vi "Loop_ProtoType Test.vi"() -> ()   [LabVIEW 2017, in "SRX SubSystem.lvlib"]
uses:
  SRX SubSystem.lvlib
  _SHARE ALL/RoboRio Share All/SRX Share All/TypeDefs SRX/Cluster_SRX_General Data.ctl
  _SHARE ALL/RoboRio Share All/SRX Share All/TypeDefs SRX/Cluster_SRX_Common Runtime Data.ctl
  _SHARE ALL/RoboRio Share All/SRX Share All/TypeDefs SRX/Cluster_SRX_Error Calculations.ctl
  _SHARE ALL/RoboRio Share All/SRX Share All/TypeDefs SRX/Cluster_SRX_Voltage Out Data.ctl
  _SHARE ALL/RoboRio Share All/SRX Share All/TypeDefs SRX/Cluster_SRX_Sensor Out Data.ctl
  _SHARE ALL/RoboRio Share All/SRX Share All/TypeDefs SRX/Cluster_SRX_Sensor Quad Data.ctl
  _SHARE ALL/RoboRio Share All/SRX Share All/TypeDefs SRX/Cluster_SRX_Analog In Data.ctl
  _SHARE ALL/RoboRio Share All/SRX Share All/TypeDefs SRX/Cluster_SRX_PWM Sensor Data.ctl
  _SHARE ALL/RoboRio Share All/SRX Share All/TypeDefs SRX/Cluster_SRX_F and R Limit Indicators.ctl
  _SHARE ALL/RoboRio Share All/SRX Share All/TypeDefs SRX/Cluster_SRX_Faults.ctl
  _SHARE ALL/RoboRio Share All/SRX Share All/TypeDefs SRX/Cluster_SRX_Config Voltage Output.ctl
  System Drivers/Phoenix-LabVIEW/Motor Controller/Controls/CTRE_Phoenix_MotorControl_NeutralMode.ctl
  _SHARE ALL/RoboRio Share All/SRX Share All/TypeDefs SRX/Cluster_SRX_Forward and Reverse.ctl
  _SHARE ALL/RoboRio Share All/SRX Share All/TypeDefs SRX/Cluster_SRX_Current Config.ctl
  _SHARE ALL/RoboRio Share All/SRX Share All/TypeDefs SRX/Cluster_SRX_Config Soft Limits.ctl
  _SHARE ALL/RoboRio Share All/SRX Share All/TypeDefs SRX/Cluster_SRX_Config Hard Limits.ctl
  System Drivers/Phoenix-LabVIEW/Motor Controller/Controls/CTRE_Phoenix_MotorControl_LimitSwitchNormal.ctl
  _SHARE ALL/RoboRio Share All/SRX Share All/TypeDefs SRX/Cluster_SRX_PIDF.ctl
  _SHARE ALL/RoboRio Share All/SRX Share All/TypeDefs SRX/Cluster_SRX_Motion Magic Config Data.ctl
  _SHARE ALL/RoboRio Share All/SRX Share All/TypeDefs SRX/Cluster_SRX_Mode and Value.ctl
  System Drivers/Phoenix-LabVIEW/Motor Controller/Controls/CTRE_Phoenix_MotorControl_ControlMode.ctl
  _SHARE ALL/RoboRio Share All/SRX Share All/TypeDefs SRX/ENUM_SRX_Reset Select.ctl
  _SHARE ALL/RoboRio Share All/SRX Share All/TypeDefs SRX/Cluster_SRX_Sensor Config.ctl
  System Drivers/Phoenix-LabVIEW/Motor Controller/Controls/CTRE_Phoenix_MotorControl_FeedbackDevice.ctl
  System Drivers/Phoenix-LabVIEW/Controls/CTRE_Phoenix_Params.ctl
  ENUM_SM_State.ctl
  <vilib>/Rock Robotics/WPI/MotorControl/WPI_MotorControlDeviceRef.ctl
  <vilib>/Rock Robotics/WPI/MotorControl/WPI_MotorControlType.ctl
  <vilib>/Rock Robotics/SystemInterfaces/DIO/FPGA_DIOPWMChannel.ctl
  <vilib>/Rock Robotics/WPI/PWM/WPI_PWMDeadband.ctl
  <vilib>/Rock Robotics/SystemInterfaces/DIO/FPGA_DIOChannel.ctl
  ENUM_SM_Action.ctl
  _SHARE ALL/Global Share All/Global_STOP.vi
  Global_CMD.vi
panel:
  out "Encoder Data":enum32{"PWM", "Analog", "Quad"}(tab)
  out "PWM Data":T1
  out "Analog Sensor Data":T2
  out "Quad Sensor Data Out":T3
  in  "TYPE":bool
  in  "Master Invert":bool
  in  "Follow Tab":T4(tab)
  in  "Follow1 Invert":bool
  in  "Follower 1":u8=14
  in  "FB Invert":bool
  in  "FA Invert":bool
  in  "Follower A":u8=14
  in  "Follower B":u8=14
  in  "Clear Error":bool
  out "Waveform Chart":cluster{"Value":dbl, "Pos":i32, "Vel":i32}(graph)
  out "Mode And Value":T5 {"Mode" items=["PercentOutput"=0, "Position"=1, "Velocity"=2, "Current"=3, "Follower"=5, "MotionProfile"=6, "MotionMagic"=7, "MotionMagicArc"=8, "MotionProfileArc"=10, "Disabled"=15]}
  out "Current Error":errorcluster
  in  "Master ID":u8=14
  in  "Tab":enum32{"Config", "Set", "Settings"}(tab)
  in  "Set Data":bool
  in  "Config":T7(tab)
  in  "Voltage Out Config":T8={"Invert?"=FALSE, "Neutral Mode"=enum."Override to Brake", "Deadband (-1to1)"=0.02, "Ramp Time Off to Full (S)"=0.01, "Peak  (-1to1)"={"Forward"=1.0, "Reverse"=-1.0}, "Nominal  (-1to1)"={"Forward"=0.0, "Reverse"=0.0}}
  in  "Sensor Config":T11={"Feedback Device"=enum."None", "PhaseSensor"=TRUE}
  in  "Current Out Config":T13
  in  "Soft Limits (Units)":T14={"Max"=200000, "Min"=-200000, "Max Enable"=TRUE, "Min Enable"=TRUE}
  in  "Hard Limits":T15
  in  "Motion Magic Config Data":T17
  in  "AllowableClosedLoopError":i32=300
  in  "Maximum I-Acc":dbl
  in  "SlotIdx":i32
  in  "Use Slot":bool
  in  "Target Slot":i32
  in  "Reset":bool
  in  "Reset Select":T18
  in  "Set PIDF 1":bool
  in  "PIDF 0":T19={"P"=0.02, "I"=0.0, "D"=6.0, "F"=0.0, "I Zone"=3000.0}
  in  "PIDF 1":T19
  in  "Set PIDF 0":bool
  in  "Enable":bool
  in  "Param Select":T20[](array[typedef]) items=["eOnBoot_BrakeMode"=31, "eQuadFilterEn"=91, "eQuadIdxPolarity"=108, "eClearPositionOnIdx"=100, "eMotionProfileHasUnderrunErr"=119, "eMotionProfileTrajectoryPointDurationMs"=120, "eClearPosOnLimitF"=144, "eClearPosOnLimitR"=145, "eStatusFramePeriod"=300, "eOpenLoopRamp"=301, "eClosedLoopRamp"=302, "eNeutralDeadband"=303, "ePeakPosOutput"=305, "eNominalPosOutput"=306, "ePeakNegOutput"=307, "eNominalNegOutput"=308, "eProfileParamSlot_P"=310, "eProfileParamSlot_I"=311, "eProfileParamSlot_D"=312, "eProfileParamSlot_F"=313, "eProfileParamSlot_IZone"=314, "eProfileParamSlot_AllowableErr"=315, "eProfileParamSlot_MaxIAccum"=316, "eClearPositionOnLimitF"=320, "eClearPositionOnLimitR"=321, "eClearPositionOnQuadIdx"=322, "eSampleVelocityPeriod"=325, "eSampleVelocityWindow"=326, "eFeedbackSensorType"=330, "eSelectedSensorPosition"=331, "eFeedbackNotContinuous"=332, "eRemoteSensorSource"=333, "eRemoteSensorDeviceID"=334, "eSensorTerm"=335, "eRemoteSensorClosedLoopDisableNeutralOnLOS"=336, "eForwardSoftLimitThreshold"=340, "eReverseSoftLimitThreshold"=341, "eForwardSoftLimitEnable"=342, "eReverseSoftLimitEnable"=343, "eNominalBatteryVoltage"=350, "eBatterVoltageFilterSize"=351, "eContinuousCurrentLimitAmps"=360, "eContinuousCurrentLimitMs"=361, "ePeakCurrentLimitAmps"=362, "eClosedLoopIAccum"=370, "eCustomParam"=380, "eStickyFaults"=390, "eAnalogPosition"=400, "eQuadraturePosition"=401, "ePulseWidthPosition"=402, "eMotMag_Accel"=410, "eMotMag_VelCruise"=411, "eLimitSwitchSource"=421, "eLimitSwitchNormClosedAndDis"=422, "eLimitSwitchDisabledNeutralOnLOS"=423, "eLimitSwitchRemoteDevID"=424]
  in  "Read Info":bool
  out "Value Array":dbl[](array[numeric])
  out "Last Error Code":i32
  out "Faults Out":T21
  out "Hard Limits":T22
  out "Last Error":errorcluster
  out "Common Runtime Data Out":T23 {"Temp" format="%.1f"; "Voltage"."Bus" format="%.3f"; "Voltage"."Output" format="%.3f"; "Voltage"."Percent" format="%.3f"; "Current" format="%.2f"}
  out "Device Info":T27
  out "Cycle Time (S)":dbl format="%.3g"
  # "VICTOR"
  # "TALON"
  # "C"
  # "Units"
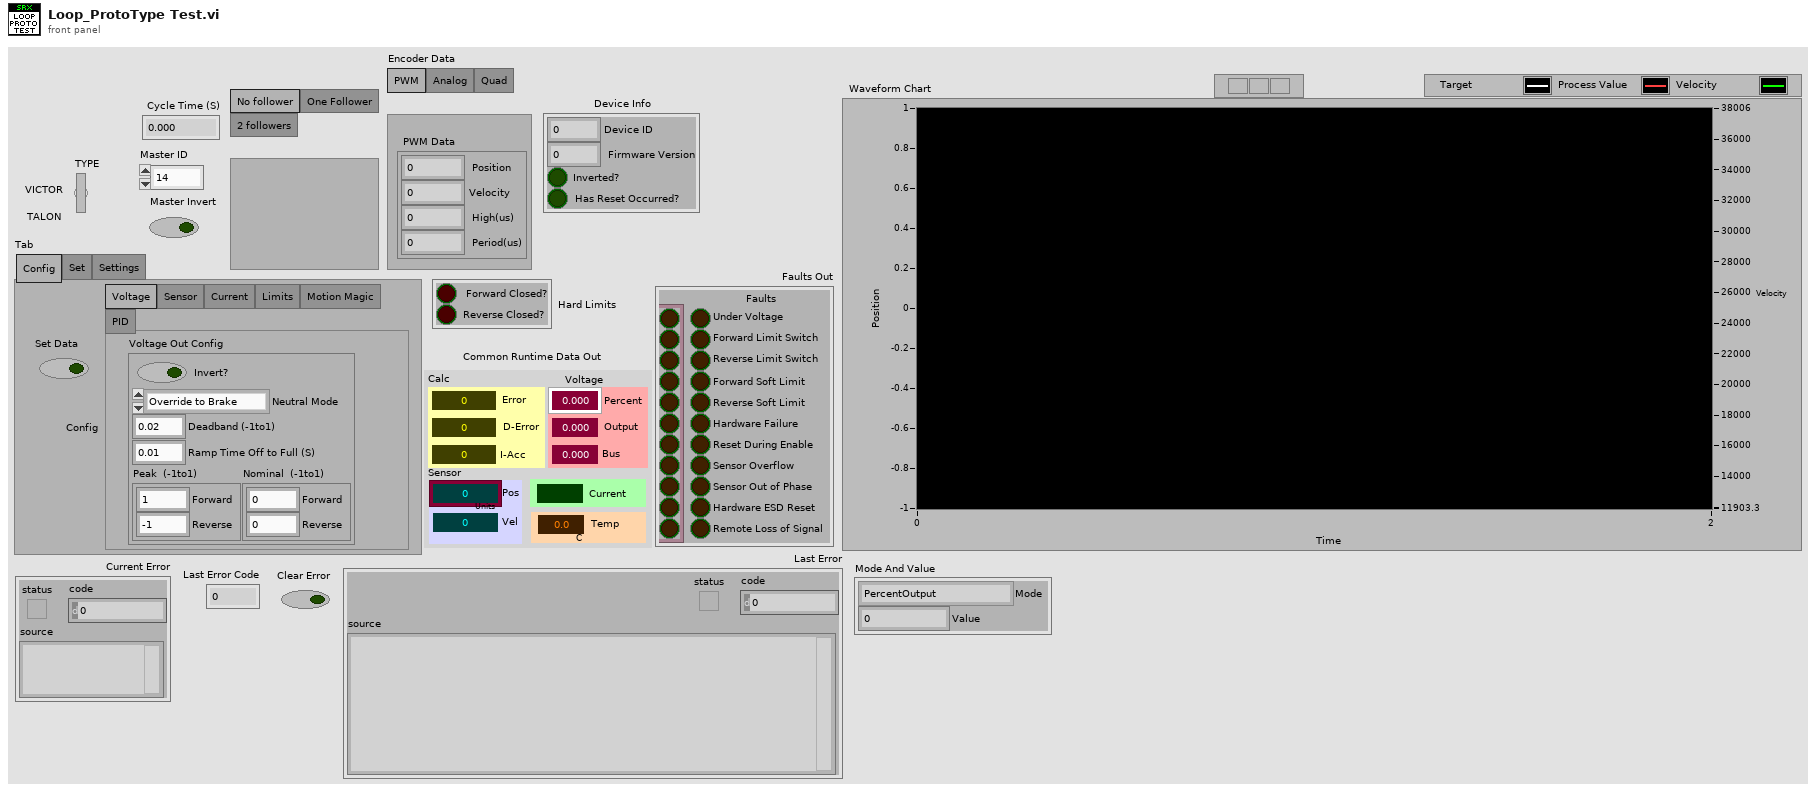
[diagram p1: front panel]
types:
  T1 = typedef "Cluster_SRX_PWM Sensor Data.ctl" = cluster{"Position":i32, "Velocity":i32, "High(us)":i32, "Period(us)":i32}
  T2 = typedef "Cluster_SRX_Analog In Data.ctl" = cluster{"WithOv":i32, "Raw":i32, "Velocity":i32}
  T3 = typedef "Cluster_SRX_Sensor Quad Data.ctl" = cluster{"Position":i32, "Velocity":i32, "Quad A Pin":bool, "Quad B Pin":bool, "Quad Idx Pin":bool}
  T4 = enum32{"No follower", "One Follower", "2 followers"}
  T5 = typedef "Cluster_SRX_Mode and Value.ctl" = cluster{"Mode":T6, "Value":dbl}
  T6 = typedef "CTRE_Phoenix_MotorControl_ControlMode.ctl" = u16
  T7 = enum32{"Voltage", "Sensor", "Current", "Limits", "Motion Magic", "PID"}
  T8 = typedef "Cluster_SRX_Config Voltage Output.ctl" = cluster{"Invert?":bool, "Neutral Mode":T9, "Deadband (-1to1)":dbl, "Ramp Time Off to Full (S)":dbl, "Peak  (-1to1)":T10, "Nominal  (-1to1)":T10}
  T9 = typedef "CTRE_Phoenix_MotorControl_NeutralMode.ctl" = enum8{"EEPROMSetting", "Override to Coast", "Override to Brake"}
  T10 = typedef "Cluster_SRX_Forward and Reverse.ctl" = cluster{"Forward":dbl, "Reverse":dbl}
  T11 = typedef "Cluster_SRX_Sensor Config.ctl" = cluster{"Feedback Device":T12, "PhaseSensor":bool}
  T12 = typedef "CTRE_Phoenix_MotorControl_FeedbackDevice.ctl" = enum16{"None", "QuadEncoder", "Analog", "Tachometer", "Pulse Width Encoded Position", "Sensor Sum (S0 + S1)", "Sensor Difference (D0 - D1)", "Remote Source 0", "Remote Source 1", "Software Emulated"}
  T13 = typedef "Cluster_SRX_Current Config.ctl" = cluster{"Enable Current Limit?":bool, "Peak Current (Amps)":i32, "Peak Current Maximum Duration (ms)":i32, "Continuous Current Limit (Amps)":i32}
  T14 = typedef "Cluster_SRX_Config Soft Limits.ctl" = cluster{"Max":i32, "Min":i32, "Max Enable":bool, "Min Enable":bool}
  T15 = typedef "Cluster_SRX_Config Hard Limits.ctl" = cluster{"Fwd Enable":bool, "Rev Enable":bool, "Fwd NO-NC":T16, "Rev NO-NC":T16}
  T16 = typedef "CTRE_Phoenix_MotorControl_LimitSwitchNormal.ctl" = enum16{"Normally Open", "Normally Closed", "Disabled"}
  T17 = typedef "Cluster_SRX_Motion Magic Config Data.ctl" = cluster{"Cruise Velocity":i32, "Acceleration":i32}
  T18 = typedef "ENUM_SRX_Reset Select.ctl" = enum16{"None", "Sensor", "I-Accum", "Sticky Faults", "ALL"}
  T19 = typedef "Cluster_SRX_PIDF.ctl" = cluster{"P":dbl, "I":dbl, "D":dbl, "F":dbl, "I Zone":dbl}
  T20 = typedef "CTRE_Phoenix_Params.ctl" = u16
  T21 = typedef "Cluster_SRX_Faults.ctl" = cluster{"Sticky":cluster{"Under Voltage":bool, "Forward Limit Switch":bool, "Reverse Limit Switch":bool, "Forward Soft Limit":bool, "Reverse Soft Limit":bool, "Hardware Failure":bool, "Reset During Enable":bool, "Sensor Overflow":bool, "Sensor Out of Phase":bool, "Hardware ESD Reset":bool, "Remote Loss of Signal":bool}, "Faults":cluster{"Under Voltage":bool, "Forward Limit Switch":bool, "Reverse Limit Switch":bool, "Forward Soft Limit":bool, "Reverse Soft Limit":bool, "Hardware Failure":bool, "Reset During Enable":bool, "Sensor Overflow":bool, "Sensor Out of Phase":bool, "Hardware ESD Reset":bool, "Remote Loss of Signal":bool}}
  T22 = typedef "Cluster_SRX_F and R Limit Indicators.ctl" = cluster{"Forward Closed?":bool, "Reverse Closed?":bool}
  T23 = typedef "Cluster_SRX_Common Runtime Data.ctl" = cluster{"Calc":T24, "Voltage ":T25, "Sensor":T26, "Current":dbl, "Temp":dbl}
  T24 = typedef "Cluster_SRX_Error Calculations.ctl" = cluster{"Error":i32, "D-Error":dbl, "I-Acc":dbl}
  T25 = typedef "Cluster_SRX_Voltage Out Data.ctl" = cluster{"Percent":dbl, "Output":dbl, "Bus":dbl}
  T26 = typedef "Cluster_SRX_Sensor Out Data.ctl" = cluster{"Pos":i32, "Vel":i32}
  T27 = typedef "Cluster_SRX_General Data.ctl" = cluster{"Device ID":i32, "Firmware Version":i32, "Inverted?":bool, "Has Reset Occurred?":bool}
  T28 = typedef "SRX SubSystem.lvlib/ENUM_SM_Action.ctl" = enum16{"No Action", "Reset Time", "Reset All", "Set Mode and Value", "Set PIDF Slot 0", "Set PIDF Slot 1", "Reset", "Set PID Slot", "Create Master SRX", "Create Followers SRX"}
  T29 = typedef "WPI_MotorControlDeviceRef.ctl" = cluster{"DeviceStatus":errorcluster, "Type":T30, "PWM":cluster{"PWM Channel":T31, "DeadBand":T32}, "CAN":cluster{"Device Number":u8, "SetOutput VI Ref":variant, "GetOutput VI Ref":variant, "Enable VI Ref":variant, "Disable VI Ref":variant, "Data":variant}, "Invert":bool, "DIO PWM":cluster{"PWM \"Enable\" Channel":T31, "DIOChannel":T33, "PWM Rate":dbl}}
  T30 = typedef "WPI_MotorControlType.ctl" = enum16{"PWM", "CAN", "DIO PWM"}
  T31 = typedef "FPGA_DIOPWMChannel.ctl" = enum8{"PWM 0", "PWM 1", "PWM 2", "PWM 3", "PWM 4", "PWM 5", "PWM 6", "PWM 7", "PWM 8", "PWM 9", "PWM MXP 0", "PWM MXP 1", "PWM MXP 2", "PWM MXP 3", "PWM MXP 4", "PWM MXP 5", "PWM MXP 6", "PWM MXP 7", "PWM MXP 8", "PWM MXP 9", "Invalid"}
  T32 = typedef "WPI_PWMDeadband.ctl" = cluster{"Name":string, "maxPositivePwm":i32, "minPositivePwm":i32, "centerPwm":i32, "maxNegativePwm":i32, "minNegativePwm":i32, "angularRange":u16}
  T33 = typedef "FPGA_DIOChannel.ctl" = enum8{"DIO 0", "DIO 1", "DIO 2", "DIO 3", "DIO 4", "DIO 5", "DIO 6", "DIO 7", "DIO 8", "DIO 9", "DIO MXP 0", "DIO MXP 1", "DIO MXP 2", "DIO MXP 3", "DIO MXP 4", "DIO MXP 5", "DIO MXP 6", "DIO MXP 7", "DIO MXP 8", "DIO MXP 9", "DIO MXP 10", "DIO MXP 11", "DIO MXP 12", "DIO MXP 13", "DIO MXP 14", "DIO MXP 15", "SPI Port CS1", "SPI Port CS2", "SPI Port CS3", "SPI Port MISO", "SPI Port MOSI", "Invalid"}
  T34 = typedef "SRX SubSystem.lvlib/ENUM_SM_State.ctl" = enum16{"Startup", "Idle", "Shutdown"}
  T35 = cluster{"State":T34, "Previous State":T34, "Current Time":timestamp, "Previous Time":timestamp, "Start Time":timestamp, "Target Time (ms)":u32, "Cycle Time(S)":dbl, "SRX Ref":T29, "Error":errorcluster, "SRX Mode":T5, "Reset Select":T18, "Target Slot":i32, "PIDF":T19, "Sensor Config":T11}
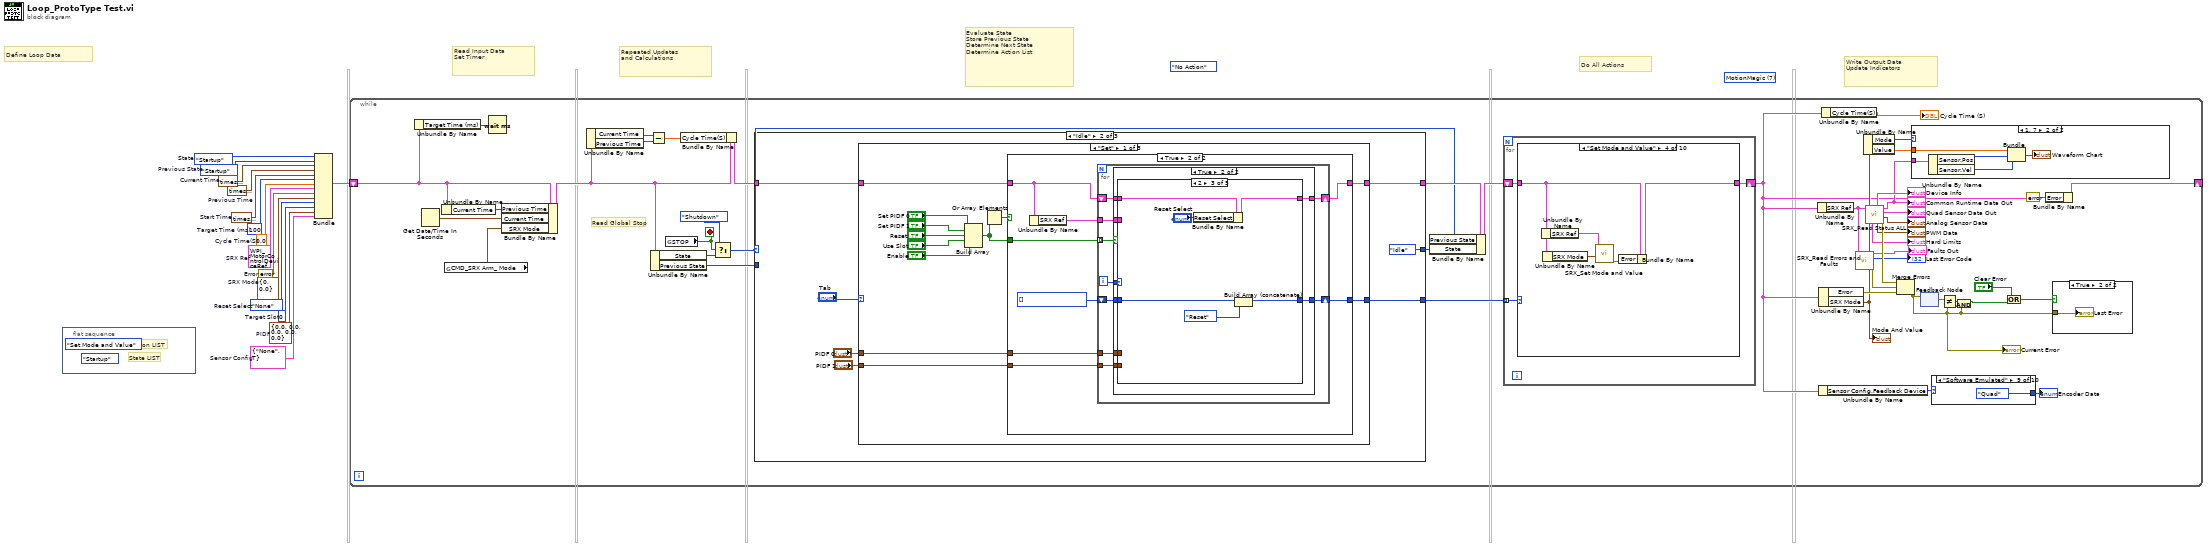
[diagram p0: block diagram]
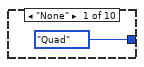
[diagram p2: hidden frame]
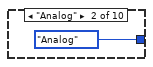
[diagram p3: hidden frame]
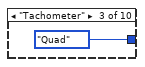
[diagram p4: hidden frame]
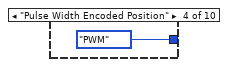
[diagram p5: hidden frame]
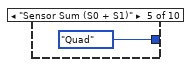
[diagram p6: hidden frame]
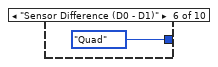
[diagram p7: hidden frame]
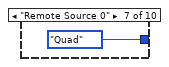
[diagram p8: hidden frame]
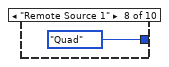
[diagram p9: hidden frame]
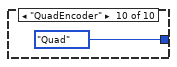
[diagram p10: hidden frame]
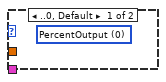
[diagram p11: hidden frame]
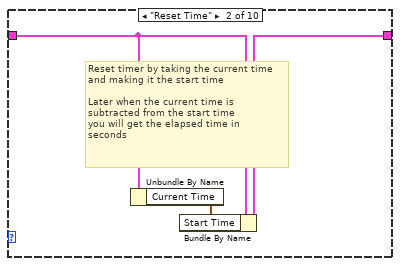
[diagram p14: hidden frame]
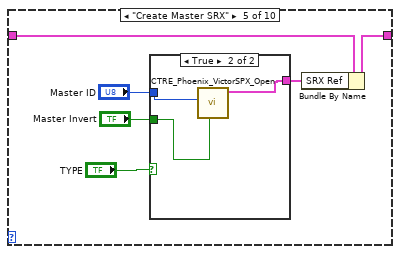
[diagram p16: hidden frame]
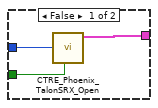
[diagram p17: hidden frame]
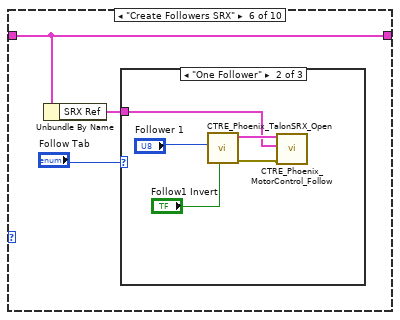
[diagram p18: hidden frame]
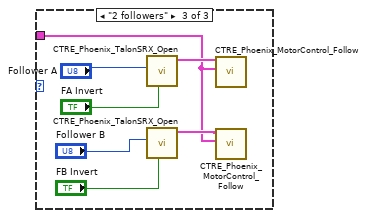
[diagram p20: hidden frame]
diagram:
  (unwired) ENUM_SM_Action."No Action" ("Action")
  w1 = T11 {"Feedback Device"=enum."None", "PhaseSensor"=TRUE}  # Sensor Config
  (unwired) T6 7 items=["PercentOutput"=0, "Position"=1, "Velocity"=2, "Current"=3, "Follower"=5, "MotionProfile"=6, "MotionMagic"=7, "MotionMagicArc"=8, "MotionProfileArc"=10, "Disabled"=15] ("Mode")
  w3 = T19 {"P"=0.0, "I"=0.0, "D"=0.0, "F"=0.0, "I Zone"=0.0}  # PIDF
  w4 = 0  # Target Slot
  w5 = ENUM_SRX_Reset_Select."None"  # Reset Select
  w6 = T5 {"Mode"=0, "Value"=0.0}  # SRX Mode
  w7 = errorcluster {"status"=FALSE, "code"=0, "source"=""}  # Error
  w8 = T29 {"DeviceStatus"={"status"=FALSE, "code"=0, "source"=""}, "Type"=enum."PWM", "PWM"={"PWM Channel"=enum."Invalid", "DeadBand"={"Name"="", "maxPositivePwm"=0, "minPositivePwm"=0, "centerPwm"=0, "maxNegativePwm"=0, "minNegativePwm"=0, "angularRange"=0}}, "CAN"={"Device Number"=0, "SetOutput VI Ref"=variant(enum8{"Percent VBus", "Current", "Speed", "Position", "Voltage"} enum."Percent VBus"), "GetOutput VI Ref"=variant(refnum<k1> refnum), "Enable VI Ref"=variant(dbl 12.0), "Disable VI Ref"=variant(enum8{"Percent VBus", "Speed", "Position", "Slave", "Unchanged / Invalid", "Voltage Compensation", "Current", "Motion Profile"} enum."Percent VBus"), "Data"=variant}, "Invert"=FALSE, "DIO PWM"={"PWM \"Enable\" Channel"=enum."Invalid", "DIOChannel"=enum."Invalid", "PWM Rate"=0.0}}  # SRX Ref
  w9 = 0.0  # Cycle Time(S)
  w10 = ENUM_SM_State."Startup"  # Previous State
  w11 = timestamp(0 s since 1904-01-01)  # Previous Time
  w12 = u32 100  # Target Time (ms)
  w13 = timestamp(0 s since 1904-01-01)  # Start Time
  w14 = timestamp(0 s since 1904-01-01)  # Current Time
  w15 = ENUM_SM_State."Startup"  # State
  # "Define Loop Data"
  # "Repeated Updates\nand Calculations"
  # "Read Input Data\nSet Timer"
  # "Evaluate State\nStore Previous State\nDetermine Next State\nDetermine Action List"
  # "Do All Actions"
  # "Write Output Data\nUpdate Indicators"
  n1 = flat-sequence {
    frame #0 {
      (unwired) ENUM_SM_State."Startup" ("State")
      (unwired) ENUM_SM_Action."Set Mode and Value" ("Action")
      # "State LIST"
      # "Action LIST"
    }
  }
  n2 = Bundle("State"=w15, "Previous State"=w10, "Current Time"=w14, "Previous Time"=w11, "Start Time"=w13, "Target Time (ms)"=w12, "Cycle Time(S)"=w9, "SRX Ref"=w8, "Error"=w7, "SRX Mode"=w6, "Reset Select"=w5, "Target Slot"=w4, "PIDF"=w3, "Sensor Config"=w1) -> (w2:T35)  [unwired: 1 in]
  n3 = while {
    shift-right: [w26] -> _
    shift-left: w2 -> [w52]
    stop <- w57 stop-if-true
    # "Read Global Stop"
    n4 = Unbundle By Name(w52) -> ("Target Time (ms)"=w54:u32)
    n5 = Get Date/Time In Seconds() -> (seconds since 1Jan1904=w61:timestamp)
    n6 = Unbundle By Name(w52) -> ("Current Time"=w53:timestamp)
    n7 = global read "Global_CMD.vi" "CMD_SRX Arm_ Mode"() -> (w42:T5)
    n8 = Wait (ms)(milliseconds to wait=w54) -> ()  [unwired: 1 out]
    n9 = Bundle By Name(cluster=w52, "Previous Time"=w53, "Current Time"=w61, "SRX Mode"=w42) -> (w46:T35)
    n10 = Unbundle By Name(w46) -> ("Current Time"=w47:timestamp, "Previous Time"=w48:timestamp)
    n11 = Subtract(x=w47, y=w48) -> (x-y=w44:dbl)
    n12 = Unbundle By Name(w46) -> ("State"=w55:T34, "Previous State"=w51:T34)
    n13 = global read "Global_STOP.vi" "STOP"() -> (w57:bool)
    n14 = Bundle By Name(cluster=w46, "Cycle Time(S)"=w44) -> (w45:T35)
    n15 = Select(t=ENUM_SM_State."Shutdown" ("State"), s=w57, f=w55) -> (s? t:f=w50:T34)
    n16 = case shown="\"Idle\"" w50 {
      tunnel: w45 -> [w140 w148 w275]
      tunnel: [w140 w147 w275] -> w59
      tunnel: [ENUM_SM_State."Idle" ("State") ENUM_SM_State."Idle" ("State") ENUM_SM_State."Shutdown" ("State")] -> w58
      tunnel: [w142 w143 w273] -> w43
      tunnel: w51 -> [_ _ _]
      frame "Startup" {
        w142 = T28[] [enum."Reset Time", enum."Create Master SRX", enum."Create Followers SRX"] items=["No Action", "Reset Time", "Reset All", "Set Mode and Value", "Set PIDF Slot 0", "Set PIDF Slot 1", "Reset", "Set PID Slot", "Create Master SRX", "Create Followers SRX"] ("Actions")
        # "E"
      }
      frame "Idle" {
        n17 = case shown="\"Set\"" "Tab" {
          tunnel: w148 -> [w155 w220 w232]
          tunnel: [w154 w220 w231] -> w147
          tunnel: "PIDF 0" -> [w152 _ w230]
          tunnel: "PIDF 1" -> [w151 _ w227]
          tunnel: [w150 _ _] -> w143
          frame "Set" {
            n18 = Build Array("Set PIDF 0", "Set PIDF 1", "Reset", "Use Slot", "Enable") -> (w153:bool[])
            n19 = Or Array Elements(Boolean array=w153) -> (logical OR=w156:bool)
            n20 = case shown="True" w156 {
              tunnel: w155 -> [w162 w166]
              tunnel: [w162 w165] -> w154
              tunnel: w153 -> [_ w170]
              tunnel: w152 -> [_ w168]
              tunnel: w151 -> [_ w167]
              tunnel: [_ w163] -> w150
              frame False {
              }
              frame True {
                w164 = T28[] [] items=["No Action", "Reset Time", "Reset All", "Set Mode and Value", "Set PIDF Slot 0", "Set PIDF Slot 1", "Reset", "Set PID Slot", "Create Master SRX", "Create Followers SRX"] ("Actions")
                n21 = Unbundle By Name(w166) -> ("SRX Ref"=w169:T29)
                n22 = for {
                  tunnel: w170 -> [w179] mode=indexing
                  tunnel: w169 -> [w178]
                  tunnel: w168 -> [w176]
                  tunnel: w167 -> [w175]
                  shift-right: [w173] -> w165
                  shift-left: w166 -> [w174]
                  shift-right: [w171] -> w163
                  shift-left: w164 -> [w172]
                  i -> [w177]
                  n23 = case shown="True" w179 {
                    tunnel: w178 -> [_ w188]
                    tunnel: w177 -> [_ w189]
                    tunnel: w176 -> [_ w187]
                    tunnel: w175 -> [_ w186]
                    tunnel: w174 -> [w181 w185]
                    tunnel: [w181 w184] -> w173
                    tunnel: w172 -> [w180 w183]
                    tunnel: [w180 w182] -> w171
                    frame False {
                    }
                    frame True {
                      n24 = case shown="2" w189 {
                        tunnel: w188 -> [_ _ _ _ _]
                        tunnel: w187 -> [w190 _ _ _ _]
                        tunnel: w186 -> [_ w196 _ _ _]
                        tunnel: w185 -> [w192 w198 w204 w213 w216]
                        tunnel: [w191 w197 w203 w212 w216] -> w184
                        tunnel: w183 -> [w195 w201 w207 w210 w217]
                        tunnel: [w194 w200 w206 w209 w215] -> w182
                        frame ..0 {
                          n25 = Bundle By Name(cluster=w192, "PIDF"=w190) -> (w191:T35)
                          n26 = Build Array (concatenate)(w195, ENUM_SM_Action."Set PIDF Slot 0" ("Action")) -> (w194:T28[])
                        }
                        frame 1 {
                          n27 = Bundle By Name(cluster=w198, "PIDF"=w196) -> (w197:T35)
                          n28 = Build Array (concatenate)(w201, ENUM_SM_Action."Set PIDF Slot 1" ("Action")) -> (w200:T28[])
                        }
                        frame 2 {
                          n29 = Bundle By Name(cluster=w204, "Reset Select"="Reset Select") -> (w203:T35)
                          n30 = Build Array (concatenate)(w207, ENUM_SM_Action."Reset" ("Action")) -> (w206:T28[])
                        }
                        frame 3 {
                          n31 = Bundle By Name(cluster=w213, "Target Slot"="Target Slot") -> (w212:T35)
                          n32 = Build Array (concatenate)(w210, ENUM_SM_Action."Set PID Slot" ("Action")) -> (w209:T28[])
                        }
                        frame 4.. {
                          n33 = Build Array (concatenate)(w217, ENUM_SM_Action."Set Mode and Value" ("Action")) -> (w215:T28[])
                        }
                      }
                    }
                  }
                }
              }
            }
          }
          frame "Settings" {
            n34 = Unbundle By Name(w220) -> ("SRX Ref"=w219:T29)
            n35 = case shown="True" "Read Info" {
              tunnel: w219 -> [_ w223]
              frame False {
              }
              frame True {
                n36 = for {
                  tunnel: w223 -> [w226]
                  tunnel: "Param Select" -> [w225] mode=indexing
                  tunnel: [w224] -> w221 mode=indexing
                  n37 = call "CTRE_Phoenix_MotorControl_ConfigGetParameter.vi"("Parameter"=w225, "PhoenixMotorControlDevRef"=w226) -> ("value"=w224:dbl)  [unwired: 7 in, 2 out]
                }
                "Value Array" <- w221
              }
            }
          }
          frame "Config" {
            n38 = case shown="True" "Set Data" {
              tunnel: w232 -> [w233 w237]
              tunnel: [w233 w236] -> w231
              tunnel: w230 -> [_ w238]
              tunnel: "Config" -> [_ w235]
              tunnel: w227 -> [_ w234]
              frame False {
              }
              frame True {
                n39 = case shown="\"Voltage\"" w235 {
                  tunnel: w238 -> [_ _ _ _ _ w272]
                  tunnel: w237 -> [w243 w246 w252 w258 w264 w271]
                  tunnel: [w242 w245 w251 w257 w263 w270] -> w236
                  tunnel: w234 -> [_ _ _ _ _ _]
                  frame "Voltage" {
                    n40 = Unbundle By Name(w243) -> ("SRX Ref"=w239:T29)
                    n41 = call "SRX_Config Voltage Output.vi"("Output Config"="Voltage Out Config", "PhoenixMotorControlDevRef"=w239) -> ("Error Out"=w241:errorcluster)  [unwired: 8 in, 1 out]
                    n42 = Bundle By Name(cluster=w243, "Error"=w241) -> (w242:T35)
                  }
                  frame "Sensor" {
                    n43 = Unbundle By Name(w246) -> ("SRX Ref"=w247:T29)
                    n44 = Bundle By Name(cluster=w246, "Sensor Config"="Sensor Config") -> (w245:T35)
                    n45 = call "SRX_Config Sensor.vi"("Sensor Config"="Sensor Config", "PhoenixMotorControlDevRef"=w247) -> ()  [unwired: 8 in, 2 out]
                  }
                  frame "Current" {
                    n46 = Unbundle By Name(w252) -> ("SRX Ref"=w250:T29)
                    n47 = call "SRX_Config Current Output.vi"("Current Config Data"="Current Out Config", "PhoenixMotorControlDevRef"=w250) -> ("Error Out"=w249:errorcluster)  [unwired: 8 in, 1 out]
                    n48 = Bundle By Name(cluster=w252, "Error"=w249) -> (w251:T35)
                  }
                  frame "Limits" {
                    n49 = Unbundle By Name(w258) -> ("SRX Ref"=w256:T29)
                    n50 = call "SRX_Config Soft Limits.vi"("Soft Limits (Units)"="Soft Limits (Units)", "PhoenixMotorControlDevRef"=w256) -> ("PhoenixMotorControlDevRef Out"=w259:T29)  [unwired: 8 in, 1 out]
                    n51 = call "SRX_Config Hard Limit Switches.vi"("Hard Limits"="Hard Limits", "PhoenixMotorControlDevRef"=w259) -> ("Error Out"=w255:errorcluster)  [unwired: 8 in, 1 out]
                    n52 = Bundle By Name(cluster=w258, "Error"=w255) -> (w257:T35)
                  }
                  frame "Motion Magic" {
                    n53 = Unbundle By Name(w264) -> ("SRX Ref"=w262:T29)
                    n54 = call "SRX_Config Motion Magic.vi"("Motion Magic Config Data"="Motion Magic Config Data", "PhoenixMotorControlDevRef"=w262) -> ("Error Out"=w261:errorcluster)  [unwired: 8 in, 1 out]
                    n55 = Bundle By Name(cluster=w264, "Error"=w261) -> (w263:T35)
                  }
                  frame "PID" {
                    n56 = Unbundle By Name(w271) -> ("SRX Ref"=w268:T29)
                    n57 = call "SRX_Config PID Closed Loop.vi"("AllowableClosedLoopError"="AllowableClosedLoopError", "SlotIdx"="SlotIdx", "Maximum Integral Accumulator Value"="Maximum I-Acc", "PIDF"=w272, "PhoenixMotorControlDevRef"=w268) -> ("Error Out"=w269:errorcluster)  [unwired: 5 in, 1 out]
                    n58 = Bundle By Name(cluster=w271, "Error"=w269) -> (w270:T35)
                  }
                }
              }
            }
          }
        }
      }
      frame "Shutdown" {
        w273 = T28[] [enum."Reset All"] items=["No Action", "Reset Time", "Reset All", "Set Mode and Value", "Set PIDF Slot 0", "Set PIDF Slot 1", "Reset", "Set PID Slot", "Create Master SRX", "Create Followers SRX"] ("Actions")
      }
    }
    n59 = Bundle By Name(cluster=w59, "Previous State"=w50, "State"=w58) -> (w60:T35)
    n60 = for {
      tunnel: w43 -> [w80] mode=indexing
      shift-right: [w79] -> w18
      shift-left: w60 -> [w78]
      n61 = case shown="\"Set Mode and Value\"" w80 {
        tunnel: w78 -> [w81 w84 w85 w87 w93 w104 w119 w125 w131 w137]
        tunnel: [w81 w83 w85 w86 w92 w104 w118 w124 w130 w136] -> w79
        frame "No Action" {
        }
        frame "Reset Time" {
          # "Reset timer by taking the current time\nand making it the start time\n\nLater when the current time is \nsubtracted from the start time\nyou will get the elapsed time in \nseconds"
          n62 = Unbundle By Name(w84) -> ("Current Time"=w82:timestamp)
          n63 = Bundle By Name(cluster=w84, "Start Time"=w82) -> (w83:T35)
        }
        frame "Reset All" {
        }
        frame "Set Mode and Value" {
          n64 = Unbundle By Name(w87) -> ("SRX Ref"=w88:T29)
          n65 = Unbundle By Name(w87) -> ("SRX Mode"=w89:T5)
          n66 = call "SRX_Set Mode and Value.vi"("Mode And Value"=w89, "PhoenixMotorControlDevRef"=w88) -> ("Error Out"=w90:errorcluster)  [unwired: 8 in, 1 out]
          n67 = Bundle By Name(cluster=w87, "Error"=w90) -> (w86:T35)
        }
        frame "Create Master SRX" {
          n68 = case shown="True" "TYPE" {
            tunnel: "Master ID" -> [w99 w102]
            tunnel: "Master Invert" -> [w98 w101]
            tunnel: [w97 w100] -> w94
            frame False {
              n69 = call "CTRE_Phoenix_TalonSRX_Open.vi"("Invert"=w98, "Device Number"=w99) -> ("CAN Talon SRX Ref"=w97:T29)  [unwired: 8 in, 1 out]
            }
            frame True {
              n70 = call "CTRE_Phoenix_VictorSPX_Open.vi"("Invert"=w101, "Device Number"=w102) -> ("CAN Talon SRX Ref"=w100:T29)  [unwired: 8 in, 1 out]
            }
          }
          n71 = Bundle By Name(cluster=w93, "SRX Ref"=w94) -> (w92:T35)
        }
        frame "Create Followers SRX" {
          n72 = Unbundle By Name(w104) -> ("SRX Ref"=w103:T29)
          n73 = case shown="\"One Follower\"" "Follow Tab" {
            tunnel: w103 -> [_ w108 w113]
            frame "No follower" {
            }
            frame "One Follower" {
              n74 = call "CTRE_Phoenix_TalonSRX_Open.vi"("Invert"="Follow1 Invert", "Device Number"="Follower 1") -> ("error out"=w107:errorcluster, "CAN Talon SRX Ref"=w109:T29)  [unwired: 8 in]
              n75 = call "CTRE_Phoenix_MotorControl_Follow.vi"("error in (no error)"=w107, "Master Controller to Follow"=w108, "PhoenixMotorControlDevRef"=w109) -> ()  [unwired: 7 in, 2 out]
            }
            frame "2 followers" {
              n76 = call "CTRE_Phoenix_TalonSRX_Open.vi"("Invert"="FA Invert", "Device Number"="Follower A") -> ("CAN Talon SRX Ref"=w117:T29)  [unwired: 8 in, 1 out]
              n77 = call "CTRE_Phoenix_TalonSRX_Open.vi"("Invert"="FB Invert", "Device Number"="Follower B") -> ("CAN Talon SRX Ref"=w115:T29)  [unwired: 8 in, 1 out]
              n78 = call "CTRE_Phoenix_MotorControl_Follow.vi"("Master Controller to Follow"=w113, "PhoenixMotorControlDevRef"=w117) -> ()  [unwired: 8 in, 2 out]
              n79 = call "CTRE_Phoenix_MotorControl_Follow.vi"("Master Controller to Follow"=w113, "PhoenixMotorControlDevRef"=w115) -> ()  [unwired: 8 in, 2 out]
            }
          }
        }
        frame "Set PIDF Slot 0" {
          n80 = Unbundle By Name(w119) -> ("SRX Ref"=w121:T29, "PIDF"=w120:T19)
          n81 = call "SRX_Set PIDF.vi"("SlotIdx"=0, "PIDF"=w120, "PhoenixMotorControlDevRef"=w121) -> ("Error Out"=w122:errorcluster)  [unwired: 7 in, 1 out]
          n82 = Bundle By Name(cluster=w119, "Error"=w122) -> (w118:T35)
        }
        frame "Set PIDF Slot 1" {
          n83 = Unbundle By Name(w125) -> ("SRX Ref"=w127:T29, "PIDF"=w126:T19)
          n84 = call "SRX_Set PIDF.vi"("SlotIdx"=1, "PIDF"=w126, "PhoenixMotorControlDevRef"=w127) -> ("Error Out"=w128:errorcluster)  [unwired: 7 in, 1 out]
          n85 = Bundle By Name(cluster=w125, "Error"=w128) -> (w124:T35)
        }
        frame "Reset" {
          n86 = Unbundle By Name(w131) -> ("SRX Ref"=w133:T29, "Reset Select"=w132:T18)
          n87 = call "SRX_Reset Select.vi"("Reset Select"=w132, "PhoenixMotorControlDevRef"=w133) -> ("Error Out"=w134:errorcluster)  [unwired: 8 in, 1 out]
          n88 = Bundle By Name(cluster=w131, "Error"=w134) -> (w130:T35)
        }
        frame "Set PID Slot" {
          n89 = Unbundle By Name(w137) -> ("SRX Ref"=w139:T29, "Target Slot"=w138:i32)
          n90 = call "CTRE_Phoenix_MotorControl_SelectProfile Slot.vi"("slotIdx"=w138, "PhoenixMotorControlDevRef"=w139) -> ("error out"=w135:errorcluster)  [unwired: 8 in, 1 out]
          n91 = Bundle By Name(cluster=w137, "Error"=w135) -> (w136:T35)
        }
      }
    }
    n92 = Unbundle By Name(w18) -> ("SRX Ref"=w41:T29)
    n93 = Unbundle By Name(w18) -> ("Sensor Config.Feedback Device"=w17:T12)
    n94 = Unbundle By Name(w18) -> ("Error"=w31:errorcluster, "SRX Mode"=w24:T5)
    "Mode And Value" <- w24
    n95 = Unbundle By Name(w18) -> ("Cycle Time(S)"=→"Cycle Time (S)":dbl)
    n96 = call "SRX_Read Errors and Faults.vi"("PhoenixMotorControlDevRef"=w41) -> ("Error Out"=w36:errorcluster, "Last Error Code Out"=→"Last Error Code":i32, "Faults Out"=→"Faults Out":T21)  [unwired: 8 in]
    n97 = Unbundle By Name(w24) -> ("Mode"=w22:T6, "Value"=w23:dbl)
    n98 = call "SRX_Read Status ALL.vi"("PhoenixMotorControlDevRef"=w41) -> ("Error Out"=w37:errorcluster, "Analog Sensor Data Out"=→"Analog Sensor Data":T2, "Quad Sensor Data Out"=→"Quad Sensor Data Out":T3, "Common Runtime Data Out"=w21:T23, "PWM Data Out"=→"PWM Data":T1, "Device Info Out"=→"Device Info":T27, "Hard Limits Out"=→"Hard Limits":T22)  [unwired: 4 in]
    "Common Runtime Data Out" <- w21
    n99 = Merge Errors(w37, w36, w31) -> (w27:errorcluster)
    "Current Error" <- w27
    n100 = case shown="1, 7" w22 {
      tunnel: w23 -> [_ w76]
      tunnel: w21 -> [_ w75]
      frame ..0, Default {
        (unwired) T6 0 items=["PercentOutput"=0, "Position"=1, "Velocity"=2, "Current"=3, "Follower"=5, "MotionProfile"=6, "MotionMagic"=7, "MotionMagicArc"=8, "MotionProfileArc"=10, "Disabled"=15] ("Mode")
      }
      frame 1, 7 {
        n101 = Unbundle By Name(w75) -> ("Sensor.Pos"=w74:i32, "Sensor.Vel"=w72:i32)
        n102 = Bundle("Value"=w76, "Pos"=w74, "Vel"=w72) -> (→"Waveform Chart":cluster{"Value":dbl, "Pos":i32, "Vel":i32})  [unwired: 1 in]
      }
    }
    n103 = feedback #1() -> (w30:errorcluster)  [unwired: 1 in]
    n104 = feedback-in #1(w27) -> ()
    n105 = case shown="\"Software Emulated\"" w17 {
      tunnel: [enum32{"PWM", "Analog", "Quad"}."Quad" ("Encoder Data") enum32{"PWM", "Analog", "Quad"}."Analog" ("Encoder Data") enum32{"PWM", "Analog", "Quad"}."Quad" ("Encoder Data") enum32{"PWM", "Analog", "Quad"}."PWM" ("Encoder Data") enum32{"PWM", "Analog", "Quad"}."Quad" ("Encoder Data") enum32{"PWM", "Analog", "Quad"}."Quad" ("Encoder Data") enum32{"PWM", "Analog", "Quad"}."Quad" ("Encoder Data") enum32{"PWM", "Analog", "Quad"}."Quad" ("Encoder Data") enum32{"PWM", "Analog", "Quad"}."Quad" ("Encoder Data") enum32{"PWM", "Analog", "Quad"}."Quad" ("Encoder Data")] -> w16
      frame "None" {
      }
      frame "Analog" {
      }
      frame "Tachometer" {
      }
      frame "Pulse Width Encoded Position" {
      }
      frame "Sensor Sum (S0 + S1)" {
      }
      frame "Sensor Difference (D0 - D1)" {
      }
      frame "Remote Source 0" {
      }
      frame "Remote Source 1" {
      }
      frame "Software Emulated" {
      }
      frame "QuadEncoder" {
      }
    }
    "Encoder Data" <- w16
    n106 = Not Equal?(x=w30, y=w27) -> (x != y?=w29:bool)
    n107 = And(x=w29, y=w27) -> (x .and. y?=w28:bool)
    n108 = Or(x="Clear Error", y=w28) -> (x .or. y?=w20:bool)
    n109 = Bundle By Name(cluster=w18, "Error"=errorcluster {"status"=FALSE, "code"=0, "source"=""}) -> (w26:T35)
    n110 = case shown="True" w20 {
      tunnel: w27 -> [_ w77]
      frame False {
      }
      frame True {
        "Last Error" <- w77
      }
    }
  }
